vi "Read Record.vi"(8 "error in (no error)":errorcluster, 10 "CSV String":string, 11 "VISA resource name":refnum<visa-resource-name>) -> (0 "error out":errorcluster, 2 "Record":dbl[](array[numeric]), 3 "VISA resource name out":refnum<visa-resource-name>)   [LabVIEW 2013, in "Watts Up Series.lvlib"]
uses:
  <instrlib>/Watts Up Series/Watts Up Series.lvlib
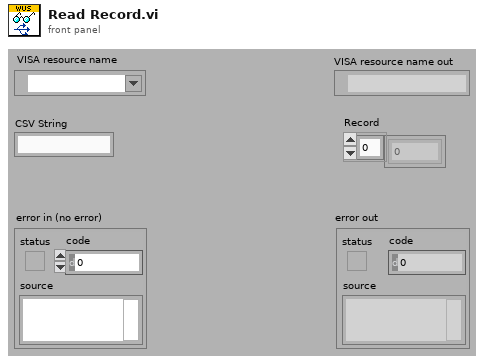
[diagram p1: front panel]
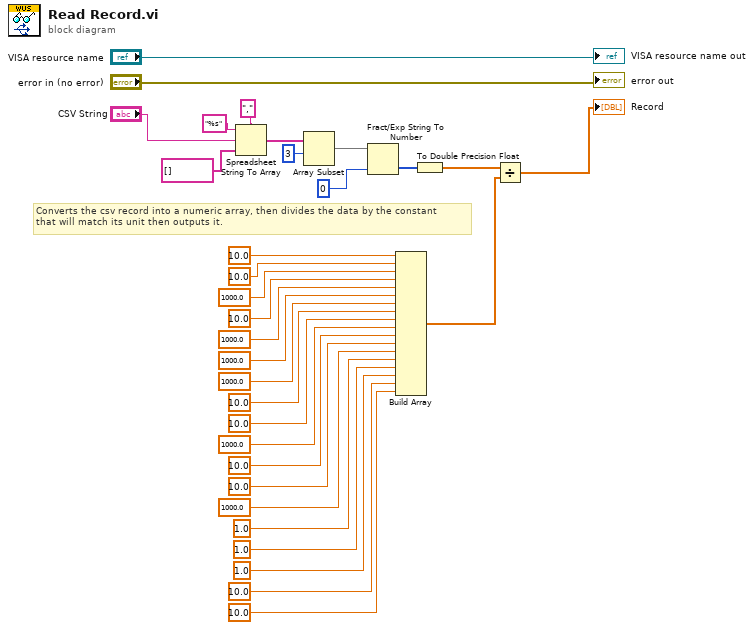
[diagram p0: block diagram]
diagram:
  # "Converts the csv record into a numeric array, then divides the data by the constant\nthat will match its unit then outputs it."
  n1 = Spreadsheet String To Array(delimiter (Tab)=",", format string="%s", spreadsheet string="CSV String", array type (2D Dbl)=string[] []) -> (array=w30:string[])
  n2 = Array Subset(array=w30, index=3) -> (w32:string[])  [unwired: 1 in]
  n3 = Fract/Exp String To Number(string=w32, default (0 dbl)=0) -> (number=w22:i32[])  [unwired: 2 in, 1 out]
  n4 = Build Array(10.0 ("element"), 10.0 ("element"), 1000.0 ("element"), 10.0 ("element"), 1000.0 ("element"), 1000.0 ("element"), 1000.0 ("element"), 10.0 ("element"), 10.0 ("element"), 1000.0 ("element"), 10.0 ("element"), 10.0 ("element"), 1000.0 ("element"), 1.0 ("element"), 1.0 ("element"), 1.0 ("element"), 10.0 ("element"), 10.0 ("element")) -> (w2:dbl[])
  n5 = To Double Precision Float(number=w22) -> (double precision float=w3:dbl[])
  n6 = Divide(x=w3, y=w2) -> (x/y=→"Record":dbl[])
  "VISA resource name out" <- "VISA resource name"
  "error out" <- "error in (no error)"
